vi "SubMarkPoint.vi"(8 "Position World":cluster{"x":sgl, "y":sgl}, 9 "Position Pixel":cluster{"x":sgl, "y":sgl}, 11 "Refnum in":T1) -> ()   [LabVIEW 2015]
uses:
  <vilib>/vision/Image Controls.llb/IMAQ Image.ctl
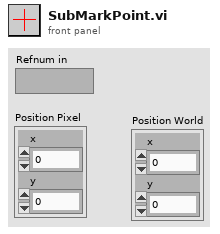
[diagram p1: front panel]
types:
  T1 = typedef "IMAQ Image.ctl" = refnum<image>
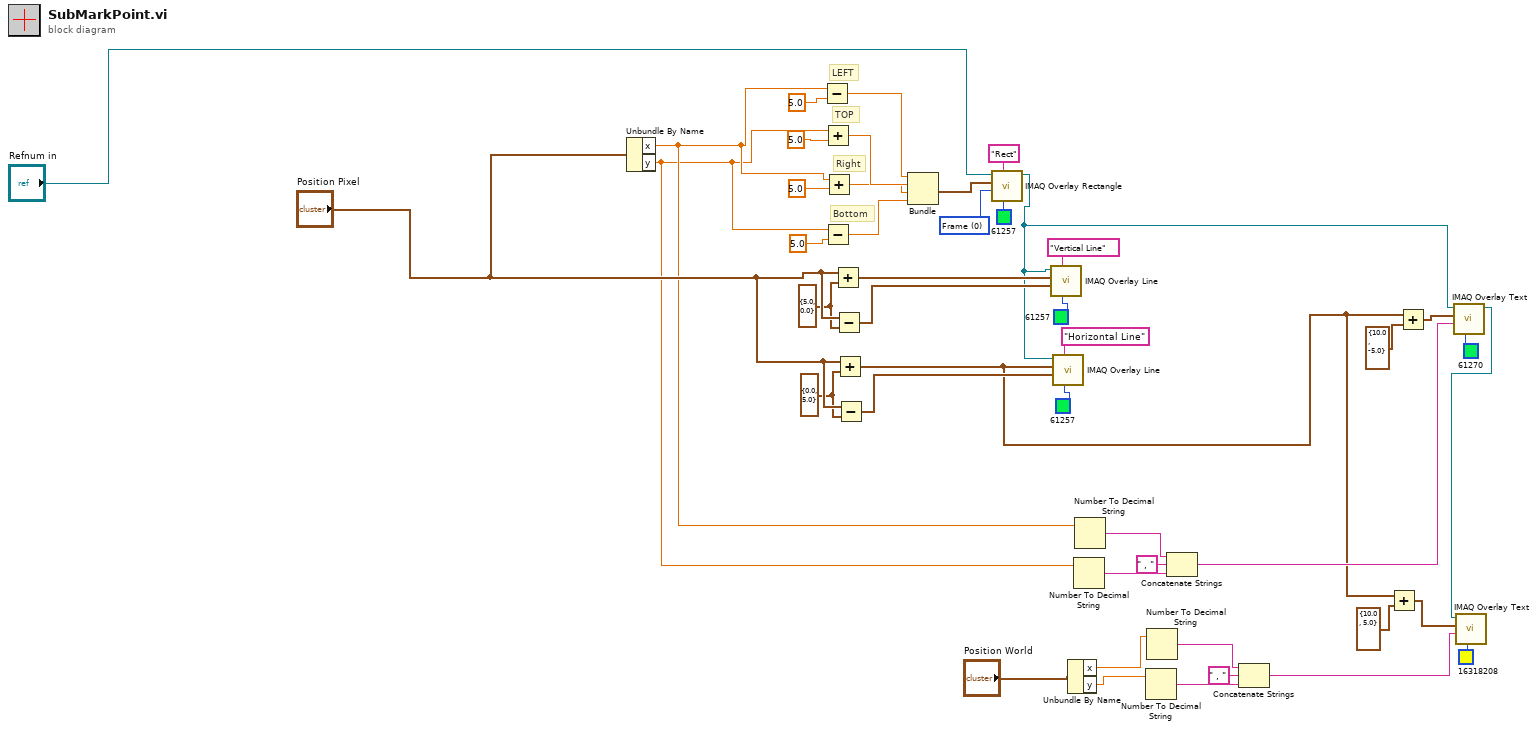
[diagram p0: block diagram]
diagram:
  w27 = cluster{"x":sgl, "y":sgl} {"x"=0.0, "y"=5.0} ("y")
  w32 = cluster{"x":sgl, "y":sgl} {"x"=5.0, "y"=0.0} ("y")
  w33 = u32 0 items=["Frame", "Fill", "Highlight"] ("Drawing Mode (Frame)")
  # "Bottom"
  # "Right"
  # "TOP"
  # "LEFT"
  n1 = Unbundle By Name("Position Pixel") -> ("x"=w19:sgl, "y"=w18:sgl)
  n2 = Subtract(x=w19, y=5.0) -> (x-y=w39:dbl)
  n3 = Add(x=w18, y=5.0) -> (x+y=w38:dbl)
  n4 = Subtract(x=w18, y=5.0) -> (x-y=w36:dbl)
  n5 = Add(x=w19, y=5.0) -> (x+y=w37:dbl)
  n6 = Add(x="Position Pixel", y=w32) -> (x+y=w23:cluster{"x":sgl, "y":sgl})
  n7 = Subtract(x="Position Pixel", y=w32) -> (x-y=w31:cluster{"x":sgl, "y":sgl})
  n8 = Add(x="Position Pixel", y=w27) -> (x+y=w1:cluster{"x":sgl, "y":sgl})
  n9 = Subtract(x="Position Pixel", y=w27) -> (x-y=w26:cluster{"x":sgl, "y":sgl})
  n10 = Bundle(w39, w38, w37, w36) -> (w35:cluster{dbl, dbl, dbl, dbl})  [unwired: 1 in]
  n11 = call "IMAQ Overlay Rectangle"("Color"=u32 61257, "Group"="Rect", "Drawing Mode (Frame)"=w33, "Rectangle"=w35, "Image"="Refnum in") -> ("Image Out"=w20:T1)  [unwired: 5 in, 1 out]
  n12 = call "IMAQ Overlay Line"("Color"=u32 61257, "Group"="Vertical Line", "End Point"=w31, "Start Point"=w23, "Image"=w20) -> ()  [unwired: 5 in, 2 out]
  n13 = call "IMAQ Overlay Line"("Color"=u32 61257, "Group"="Horizontal Line", "End Point"=w26, "Start Point"=w1, "Image"=w20) -> ()  [unwired: 5 in, 2 out]
  n14 = Unbundle By Name("Position World") -> ("x"=w9:sgl, "y"=w8:sgl)
  n15 = Number To Decimal String(number=w18) -> (decimal integer string=w16:string)  [unwired: 1 in]
  n16 = Number To Decimal String(number=w19) -> (decimal integer string=w17:string)  [unwired: 1 in]
  n17 = Number To Decimal String(number=w8) -> (decimal integer string=w11:string)  [unwired: 1 in]
  n18 = Number To Decimal String(number=w9) -> (decimal integer string=w12:string)  [unwired: 1 in]
  n19 = Concatenate Strings(w17, " , " ("string"), w16) -> (w14:string)
  n20 = Concatenate Strings(w12, " , " ("string"), w11) -> (w6:string)
  n21 = Add(x=w1, y=cluster{"x":sgl, "y":sgl} {"x"=10.0, "y"=5.0}) -> (x+y=w3:cluster{"x":sgl, "y":sgl})
  n22 = Add(x=w1, y=cluster{"x":sgl, "y":sgl} {"x"=10.0, "y"=-5.0}) -> (x+y=w21:cluster{"x":sgl, "y":sgl})
  n23 = call "IMAQ Overlay Text"("Text Color (black)"=u32 61270, "String"=w14, "Origin"=w21, "Image"=w20) -> ("Image Out"=w7:T1)  [unwired: 6 in, 1 out]
  n24 = call "IMAQ Overlay Text"("Text Color (black)"=u32 16318208, "String"=w6, "Origin"=w3, "Image"=w7) -> ()  [unwired: 6 in, 2 out]
